vi "LitePoint_VSAConfig_PowerFreq.vi"(7 "Transmission":u16(ring) items=["CW", "Waveform"], 8 "error in (no error)":errorcluster, 9 "Power":dbl, 10 "Freq_MHz":dbl=3500.0, 11 "VISA resource name":refnum<visa-resource-name>="LitePoint_IQxstream") -> (0 "error out":errorcluster, 3 "VISA resource name out":refnum<visa-resource-name>="LitePoint_IQxstream")   [LabVIEW 2020, in "LitePoints.lvlib"]
uses:
  LitePoints.lvlib
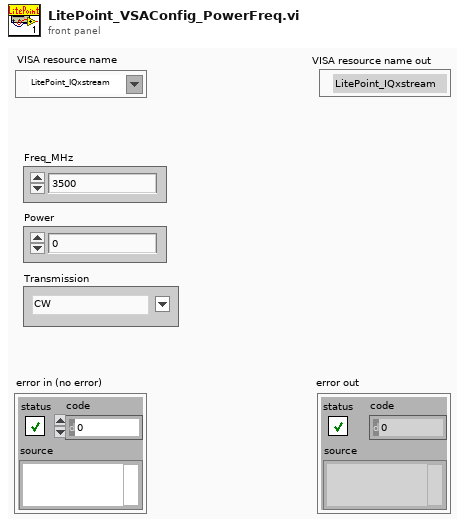
[diagram p1: front panel]
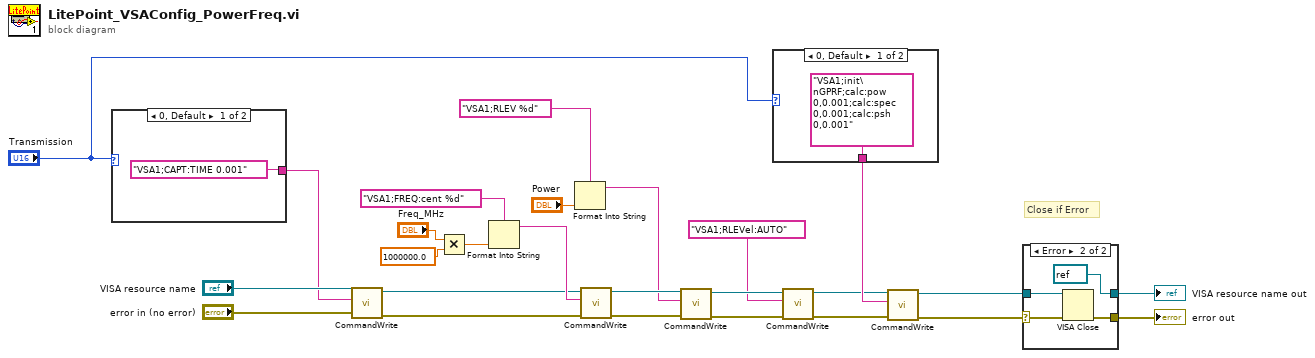
[diagram p0: block diagram]
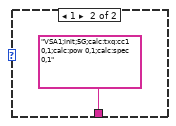
[diagram p2: hidden frame]
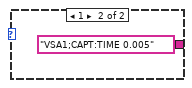
[diagram p3: hidden frame]
diagram:
  # "Close if Error"
  n1 = case shown="0, Default" "Transmission" {
    tunnel: ["VSA1;CAPT:TIME 0.001" "VSA1;CAPT:TIME 0.005"] -> w10
    frame 0, Default {
    }
    frame 1 {
    }
  }
  n2 = call "CommandWrite.vi"("error in (no error)"="error in (no error)", "Write Buffer"=w10, "VISA resource name"="VISA resource name") -> ("error out"=w12:errorcluster, "VISA resource name out"=w13:refnum<visa-resource-name>)  [unwired: 7 in]
  n3 = Multiply(x="Freq_MHz", y=1000000.0) -> (x*y=w18:dbl)
  n4 = Format Into String(format string="VSA1;FREQ:cent %d", w18) -> (resulting string=w19:string)  [unwired: 2 in, 1 out]
  n5 = Format Into String(format string="VSA1;RLEV %d", "Power") -> (resulting string=w21:string)  [unwired: 2 in, 1 out]
  n6 = call "CommandWrite.vi"("error in (no error)"=w12, "Write Buffer"=w19, "VISA resource name"=w13) -> ("error out"=w23:errorcluster, "VISA resource name out"=w24:refnum<visa-resource-name>)  [unwired: 7 in]
  n7 = call "CommandWrite.vi"("error in (no error)"=w23, "Write Buffer"=w21, "VISA resource name"=w24) -> ("error out"=w5:errorcluster, "VISA resource name out"=w4:refnum<visa-resource-name>)  [unwired: 7 in]
  n8 = case shown="0, Default" "Transmission" {
    tunnel: ["VSA1;init\nGPRF;calc:pow 0,0.001;calc:spec 0,0.001;calc:psh 0,0.001" "VSA1;init;5G;calc:txq:cc1 0,1;calc:pow 0,1;calc:spec 0,1"] -> w7
    frame 0, Default {
    }
    frame 1 {
    }
  }
  n9 = call "CommandWrite.vi"("error in (no error)"=w5, "Write Buffer"="VSA1;RLEVel:AUTO", "VISA resource name"=w4) -> ("error out"=w2:errorcluster, "VISA resource name out"=w3:refnum<visa-resource-name>)  [unwired: 7 in]
  n10 = call "CommandWrite.vi"("error in (no error)"=w2, "Write Buffer"=w7, "VISA resource name"=w3) -> ("error out"=w8:errorcluster, "VISA resource name out"=w9:refnum<visa-resource-name>)  [unwired: 7 in]
  n11 = case shown="Error" w8 {
    selector: w8 -> [w31 w34]
    tunnel: w9 -> [w32 w35]
    tunnel: [w32 refnum<visa-resource-name> refnum ("VISA resource name out")] -> w26
    tunnel: [w31 w33] -> w25
    frame No Error {
    }
    frame Error {
      n12 = VISA Close(VISA resource name=w35, error in (no error)=w34) -> (error out=w33:errorcluster)
    }
  }
  "VISA resource name out" <- w26
  "error out" <- w25
